vi "test_scd_IsDeviceBusy.vi"(8 "error in":errorcluster, 11 "SCD in":refnum<class "SCD.lvclass">) -> (0 "error out":errorcluster, 3 "SCD out":refnum<class "SCD.lvclass">)   [LabVIEW 2023, in "horiba.test.lvlib"]
uses:
  Classes/SCD/SCD.lvclass
  <vilib>/addons/_JKI Toolkits/Caraya/classes/Assert/Assert False.vi
  horiba.test.lvlib
  <vilib>/addons/_JKI Toolkits/Caraya/classes/Test/Test.lvclass
  <vilib>/addons/_JKI Toolkits/Caraya/classes/Assert/Assert.lvclass
  <userlib>/_OpenG.lib/lvdata/lvdata.llb/openg_variant.lvlib
panel:
  # "Connector Pane"
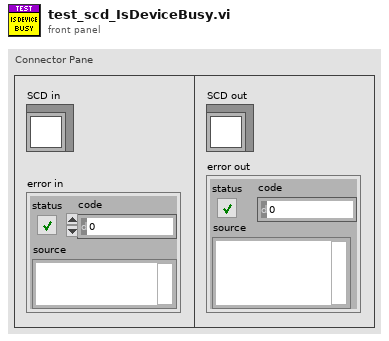
[diagram p1: front panel]
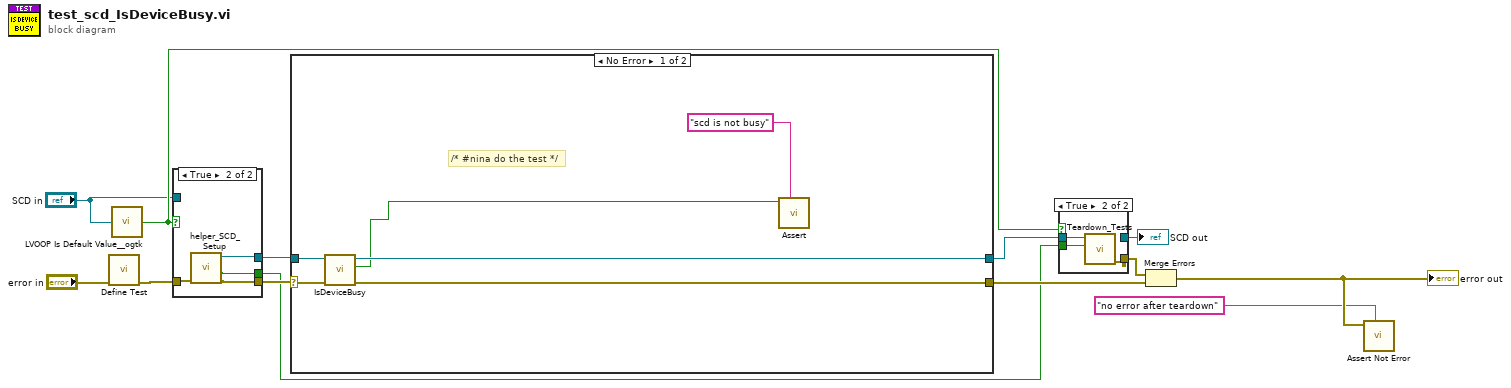
[diagram p0: block diagram]
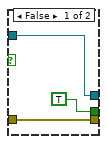
[diagram p3: hidden frame]
diagram:
  n1 = call <vilib>:"Define Test.vi"("error in (no error)"="error in") -> ("error out"=w9:errorcluster)  [unwired: 9 in, 1 out]
  n2 = call <userlib>:"LVOOP Is Default Value__ogtk.vi"("Object"="SCD in") -> ("Is Default Value?"=w3:bool)
  n3 = case shown="True" w3 {
    tunnel: w9 -> [w16 w18]
    tunnel: [w16 w20] -> w8
    tunnel: [w14 w17] -> w7
    tunnel: [TRUE ("Module Was Already Running?") w19] -> w4
    tunnel: "SCD in" -> [w14 _]
    frame False {
    }
    frame True {
      n4 = call "helper_SCD_Setup.vi"("error in"=w18) -> ("error out"=w20:errorcluster, "Module Was Already Running?"=w19:bool, "SCD out"=w17:refnum<class "SCD.lvclass">)  [unwired: 7 in, 1 out]
    }
  }
  n5 = case shown="No Error" w8 {
    selector: w8 -> [w25 w28]
    tunnel: [w23 w27] -> w12
    tunnel: w7 -> [w26 w27]
    tunnel: [w22 w28] -> w11
    frame No Error {
      # "/* #nina do the test */"
      n6 = call "IsDeviceBusy.vi"("error in (no error)"=w25, "SCD in"=w26) -> ("error out"=w22:errorcluster, "isBusy"=w21:bool, "SCD out"=w23:refnum<class "SCD.lvclass">)  [unwired: 7 in]
      n7 = call-poly <vilib>:"Assert.vi"("Label"="scd is not busy", "False?"=w21) -> ()  [unwired: 8 in, 2 out]
    }
    frame Error {
    }
  }
  n8 = case shown="True" w3 {
    tunnel: w12 -> [w29 w32]
    tunnel: [_ w31] -> w6
    tunnel: w4 -> [_ w30]
    tunnel: [w29 _] -> w1
    frame False {
    }
    frame True {
      n9 = call "Teardown_Tests.vi"("Module Was Already Running?"=w30, "horiba.lvlib:GenericDevice"=w32) -> ("error out"=w31:errorcluster)  [unwired: 8 in, 1 out]
    }
  }
  "SCD out" <- w1
  n10 = Merge Errors(w6, w11) -> (w10:errorcluster)
  "error out" <- w10
  n11 = call <vilib>:"Assert Not Error.vi"("Label"="no error after teardown", "Not Error?"=w10) -> ()  [unwired: 8 in, 2 out]
